vi "setFPGA.vi"(10 "FPGA":refnum<class "FPGA.lvclass">, 11 "HealthAndStatusDataFIFO in":refnum<class "HealthAndStatusDataFIFO.lvclass">) -> (3 "HealthAndStatusDataFIFO out":refnum<class "HealthAndStatusDataFIFO.lvclass">)   [LabVIEW 2016, in "HealthAndStatusDataFIFO.lvclass"]
uses:
  HealthAndStatusDataFIFO.lvclass
  FPGA/FPGA.lvclass
  HealthAndStatusDataFIFO.lvclass/HealthAndStatusDataFIFO.ctl
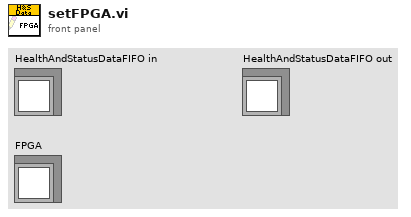
[diagram p1: front panel]
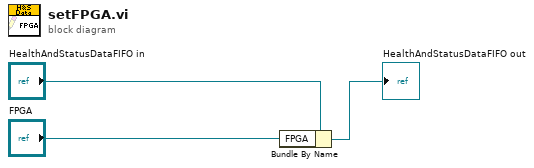
[diagram p0: block diagram]
diagram:
  n1 = Bundle By Name(cluster="HealthAndStatusDataFIFO in", "FPGA"="FPGA") -> (→"HealthAndStatusDataFIFO out":refnum<class "HealthAndStatusDataFIFO.lvclass">)
